vi "niFPGA BFGroup Input Buffer 64 U32.vi"(0 "data in":u32=8, 1 "reset":bool) -> (4 "x out":u32, 6 "y out":u32 max=0)   [LabVIEW 2017]
uses:
  <vilib>/Utility/error.llb/Clear Errors.vi
  <vilib>/rvi/Emulation/niFpgaSctlEmulationGetInTimedLoop.vi
  <vilib>/rvi/DataTransferAndStorage/Container/Common/niFpgaContainerGetUniqueNameForEmu.vi
  <vilib>/rvi/DataTransferAndStorage/Container/Common/niFpgaContainerSetEmuInfo.vi
  <vilib>/rvi/eio/common/nirviEmuReportErrorAndStop.vi
  <vilib>/rvi/Memory/Memory_Emulation/nirvimemoryEmulation.vi
  <vilib>/rvi/Memory/Memory_Emulation/nirvimemoryFastEmulation.vi
  <vilib>/rvi/Memory/Memory_Emulation/niFpgaMemoryEmulationCacheClearOnFirstRun.vi
  <vilib>/rvi/Memory/Memory_Emulation/nirvimemoryEmulationManagerCache_MakeExclusive.vi
  <vilib>/rvi/Memory/Memory_Emulation/niFpgaMemoryEmulationValidateCache.vi
  <vilib>/rvi/Memory/Memory_Emulation/nirvimemoryEmulationManagerCache_InsertValue.vi
  <vilib>/rvi/Memory/Memory_Emulation/nirvimemoryEmulationManagerCache_ReleaseExclusive.vi
  <vilib>/rvi/Memory/Memory_Emulation/nirvimemoryEmulationManagerCache_GetValue.vi
  <vilib>/rvi/Emulation/niFpgaEmulationIsFPGAContextNoSignature.vi
  <vilib>/rvi/Memory/Memory_Emulation/nirvimemoryEmulationManagerCache_SetValue.vi
  <vilib>/rvi/Emulation/niFpgaSctlEmulationResourceMgr.vi
  <vilib>/rvi/LocalResourceManager/LocalResourceManager.xnode
  <vilib>/rvi/DataTransferAndStorage/Container/XNode/niFpgaContainer.xnode
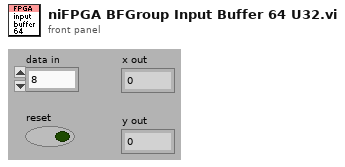
[diagram p1: front panel]
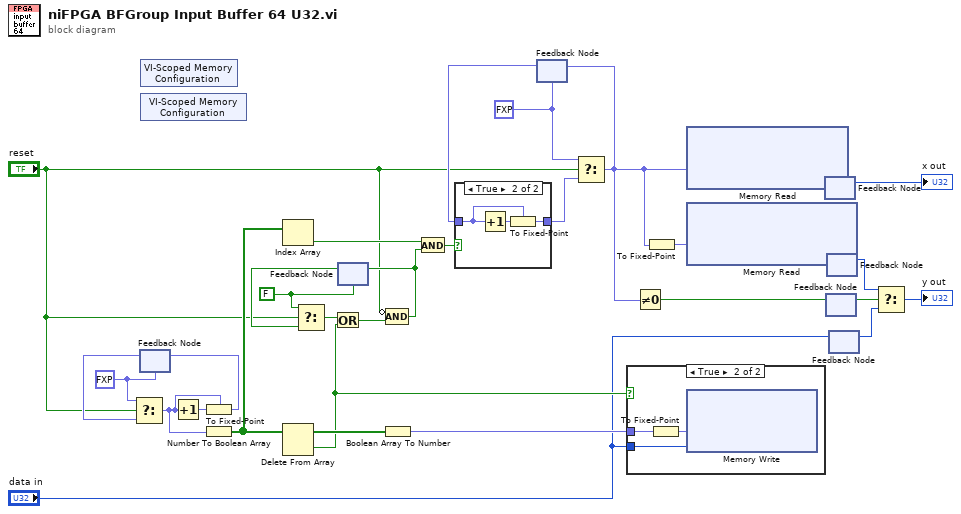
[diagram p0: block diagram]
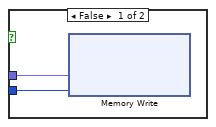
[diagram p3: hidden frame]
diagram:
  w20 = fxp<+,5,5> 0.0
  w11 = FALSE
  w25 = fxp<+,6,6> 63.0
  n1 = feedback #1(w25) -> (w31:fxp<+,6,6>)
  n2 = Select(t=w25, s="reset", f=w31) -> (s? t:f=w6:fxp<+,6,6>)
  n3 = xnode "VI-Scoped Memory Configuration"() -> ()  [unwired: 1 out]
  n4 = xnode "VI-Scoped Memory Configuration"() -> ()  [unwired: 1 out]
  n5 = Increment(x=w6) -> (x+1=w8:fxp<+,7,7>)
  n6 = To Fixed-Point(fixed-point type=w6, number=w8) -> (fixed-point=w7:fxp<+,6,6>)
  n7 = feedback-in #1(w7) -> ()
  n8 = Number To Boolean Array(number=w6) -> (Boolean array=w26:bool[])
  n9 = Index Array(array=w26) -> (element=w30:bool)  [unwired: 1 in]
  n10 = Delete From Array(array=w26) -> (deleted portion=w28:bool, array with subset deleted=w29:bool[])  [unwired: 2 in]
  n11 = feedback #2(w11) -> (w5:bool)
  n12 = Select(t=w11, s="reset", f=w5) -> (s? t:f=w12:bool)
  n13 = Or(x=w12, y=w28) -> (x .or. y?=w10:bool)
  n14 = Boolean Array To Number(Boolean array=w29) -> (number=w27:fxp<+,5,5>)
  n15 = Compound Arithmetic op=AND(invert "reset", w10) -> (w9:bool)
  n16 = feedback-in #2(w9) -> ()
  n17 = And(x=w30, y=w9) -> (x .and. y?=w22:bool)
  n18 = feedback #3(w20) -> (w24:fxp<+,5,5>)
  n19 = case shown="True" w22 {
    tunnel: w24 -> [w32 w33]
    tunnel: [w32 w34] -> w23
    frame False {
    }
    frame True {
      n20 = Increment(x=w33) -> (x+1=w35:fxp<+,6,6>)
      n21 = To Fixed-Point(fixed-point type=w33, number=w35) -> (fixed-point=w34:fxp<+,5,5>)
    }
  }
  n22 = Select(t=w20, s="reset", f=w23) -> (s? t:f=w1:fxp<+,5,5>)
  n23 = feedback-in #3(w1) -> ()
  n24 = case shown="True" w28 {
    tunnel: "data in" -> [w37 w40]
    tunnel: w27 -> [w36 w39]
    frame False {
      n25 = xnode ("Memory Write")("Address"=w36, "Data"=w37) -> ()  [unwired: 2 out]
    }
    frame True {
      n26 = To Fixed-Point(number=w39) -> (fixed-point=w38:fxp<+,4,4>)  [unwired: 1 out]
      n27 = xnode ("Memory Write")("Address"=w38, "Data"=w40) -> ()  [unwired: 2 out]
    }
  }
  n28 = Not Equal To 0?(x=w1) -> (x != 0?=w3:bool)
  n29 = To Fixed-Point(number=w1) -> (fixed-point=w13:fxp<+,4,4>)  [unwired: 1 out]
  n30 = xnode ("Memory Read")("Address"=w1) -> ("Data"=w19:u32)  [unwired: 2 out]
  n31 = xnode ("Memory Read")("Address"=w13) -> ("Data"=w14:u32)  [unwired: 2 out]
  n32 = feedback-in #4(w19) -> ()
  n33 = feedback #4() -> (→"x out":u32)  [unwired: 1 out]
  n34 = feedback-in #5(w3) -> ()
  n35 = feedback #5() -> (w2:bool)  [unwired: 1 out]
  n36 = feedback-in #6(w14) -> ()
  n37 = feedback #6() -> (w18:u32)  [unwired: 1 out]
  n38 = feedback-in #7("data in") -> ()
  n39 = feedback #7() -> (w16:u32)  [unwired: 1 out]
  n40 = Select(t=w18, s=w2, f=w16) -> (s? t:f=→"y out":u32)
